vi "Thermal_Test_SubVi_datatostring.vi"(11 "Data":dbl[](array[numeric])) -> (2 "String":string, 3 "String 3":string)   [LabVIEW 2020]
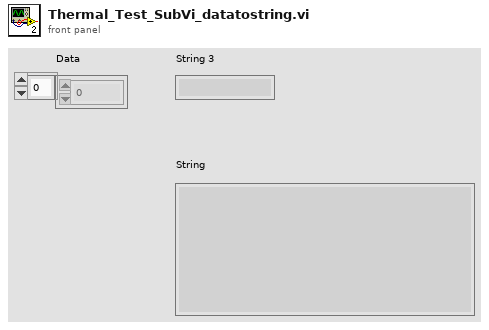
[diagram p1: front panel]
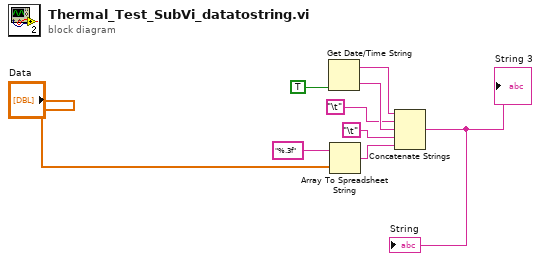
[diagram p0: block diagram]
diagram:
  n1 = Get Date/Time String(want seconds? (F)=TRUE) -> (date string=w2:string, time string=w3:string)  [unwired: 2 in]
  n2 = Array To Spreadsheet String(array="Data", 3:"%.3f") -> (spreadsheet string=w5:string)  [unwired: 1 out]
  n3 = Concatenate Strings(w2, "\t" ("Tab"), w3, "\t" ("Tab"), w5) -> (→"String" →"String 3":string)
